vi "Analog to LCD 16x2.vi"   [LabVIEW 2014]
uses:
  <vilib>/Aledyne-TSXperts/Arduino Compatible Compiler for LabVIEW/Code Generator/Arduino APIs/I2C LCD/LiquidCrystal_I2C write String.vi
  <vilib>/Aledyne-TSXperts/Arduino Compatible Compiler for LabVIEW/Arduino Compatible Compiler for LabVIEW.lvlib
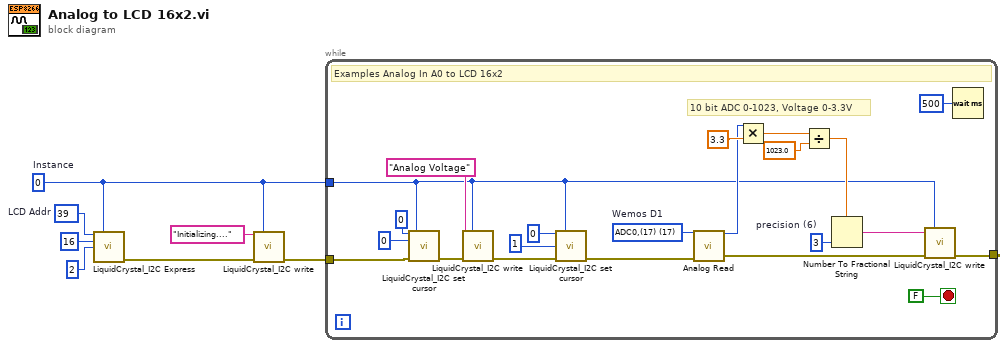
[diagram p0: block diagram]
diagram:
  w5 = u8 39  # LCD Addr
  w1 = u8 0  # Instance
  n1 = call <vilib>:"LiquidCrystal_I2C Express.vi"("Addr"=w5, "Instance"=w1, "Chars"=u16 16, "Lines"=u16 2) -> ("error out"=w4:errorcluster)  [unwired: 11 in]
  n2 = call-poly <vilib>:"LiquidCrystal_I2C write.vi"("Data"="Initializing....", "Instance"=w1, "error in (no error)"=w4) -> ("error out"=w2:errorcluster)  [unwired: 12 in]
  n3 = while {
    tunnel: w2 -> [w18]
    tunnel: w1 -> [w13]
    tunnel: [w10] -> _
    stop <- FALSE stop-if-true
    w8 = u8 17 items=["D0-RX(3)"=3, "D1-TX(1)"=1, "D2(16)"=16, "D3/D15/SCL(5)"=5, "D4/D14/SDA(4)"=4, "D5/D13/SCK(14)-(LED)"=14, "D6/D12/MISO(12)"=12, "D7/D11/MOSI(13)"=13, "D8(0)"=0, "D9/TX1(2)"=2, "D10/SS (15)"=15, "ADC0,(17)"=17]  # Wemos D1
    w23 = i16 3  # precision (6)
    # "10 bit ADC 0-1023, Voltage 0-3.3V"
    # "Examples Analog In A0 to LCD 16x2"
    n4 = call <vilib>:"LiquidCrystal_I2C set cursor.vi"("character"=u16 0, "Instance"=w13, "line"=u16 0, "error in (no error)"=w18) -> ("error out"=w19:errorcluster)  [unwired: 11 in]
    n5 = call-poly <vilib>:"LiquidCrystal_I2C write.vi"("Data"="Analog Voltage", "Instance"=w13, "error in (no error)"=w19) -> ("error out"=w16:errorcluster)  [unwired: 12 in]
    n6 = call <vilib>:"LiquidCrystal_I2C set cursor.vi"("character"=u16 0, "Instance"=w13, "line"=u16 1, "error in (no error)"=w16) -> ("error out"=w15:errorcluster)  [unwired: 11 in]
    n7 = call <vilib>:"Analog Read.vi"("pin"=w8, "error in (no error)"=w15) -> ("data"=w21:u16, "error out"=w12:errorcluster)  [unwired: 12 in]
    n8 = Multiply(x=w21, y=3.3) -> (x*y=w25:dbl)
    n9 = Divide(x=w25, y=1023.0 ("x")) -> (x/y=w22:dbl)
    n10 = Number To Fractional String ("Number To String")(number=w22, precision (6)=w23) -> (F-format string=w14:string)  [unwired: 2 in]
    n11 = call-poly <vilib>:"LiquidCrystal_I2C write.vi"("Data"=w14, "Instance"=w13, "error in (no error)"=w12) -> ("error out"=w10:errorcluster)  [unwired: 12 in]
    n12 = Wait (ms)(milliseconds to wait=u32 500) -> ()  [unwired: 1 out]
  }
